vi "Shutdown HW.vi"(8 "error in (no error)":errorcluster, 11 "DAQmx Switch in":refnum<class "DAQmx Switch.lvclass">) -> (0 "error out":errorcluster, 3 "DAQmx Switch out":refnum<class "DAQmx Switch.lvclass">)   [LabVIEW 2020, in "DAQmx Switch.lvclass"]
uses:
  DAQmx Switch.lvclass
  DAQmx Switch.lvclass/DAQmx Switch.ctl
  Switch.lvclass
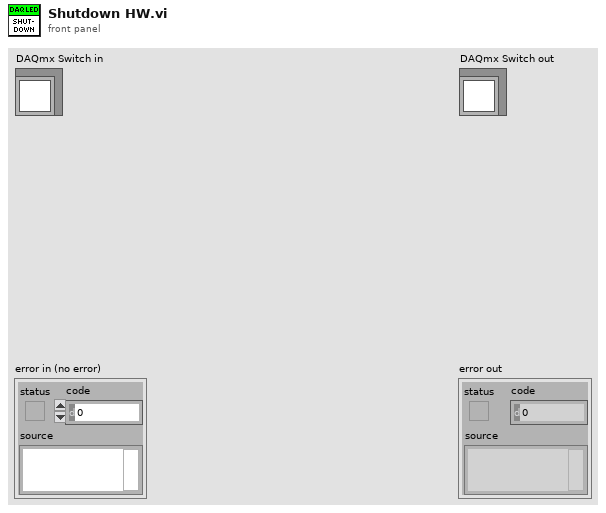
[diagram p1: front panel]
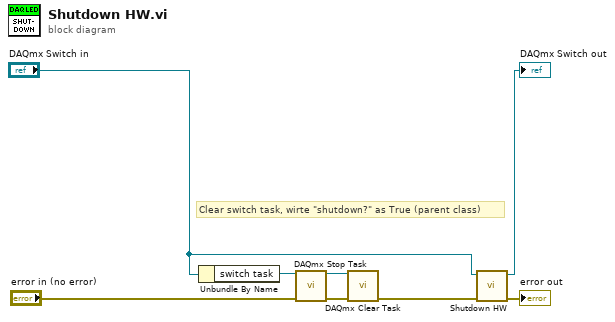
[diagram p0: block diagram]
diagram:
  # "Clear switch task, wirte \"shutdown?\" as True (parent class)"
  n1 = Unbundle By Name("DAQmx Switch in") -> ("switch task"=w3:refnum<k21>)
  n2 = call <vilib>:"DAQmx Stop Task.vi"("task/channels in"=w3, "error in"="error in (no error)") -> ("task out"=w2:refnum<k21>, "error out"=w5:errorcluster)  [unwired: 12 in]
  n3 = call <vilib>:"DAQmx Clear Task.vi"("task in"=w2, "error in"=w5) -> ("error out"=w4:errorcluster)  [unwired: 13 in]
  n4 = call-parent "Shutdown HW.vi"("error in (no error)"=w4, "Switch in"="DAQmx Switch in") -> ("error out"=→"error out":errorcluster, "Switch out"=→"DAQmx Switch out":refnum<class "DAQmx Switch.lvclass">)  [unwired: 8 in]
